vi "Example Write.vi"() -> ()   [LabVIEW 2010]
uses:
  C:/tf/play/labview/Tinkerforge.dll
  Tinkerforge.dll
panel:
  in  "stop":bool
  in  "uid":string="5556"
  in  "port":i32=4223
  in  "host":string="localhost"
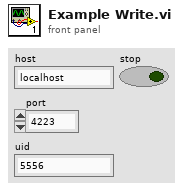
[diagram p1: front panel]
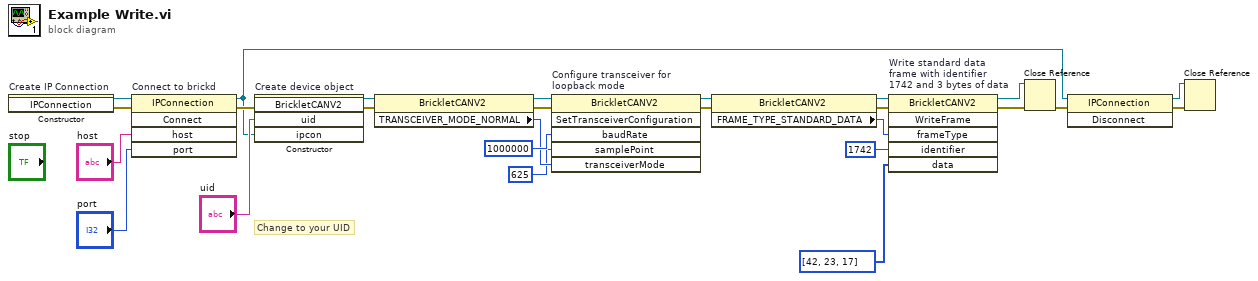
[diagram p0: block diagram]
diagram:
  # "Change to your UID"
  n1 = constructor on="Create IP Connection" class="IPConnection"() -> (reference out=w26:refnum<k24>, error out=w17:errorcluster)  [unwired: 3 in, 1 out]
  n2 = invoke on="Connect to brickd" class="IPConnection" method="Connect"(reference=w26, error in=w17, "host"="host", "port"="port") -> (reference out=w19:refnum<k24>, error out=w22:errorcluster)  [unwired: 1 in, 3 out]
  n3 = constructor on="Create device object" class="BrickletCANV2"(error in=w22, "uid"="uid", "ipcon"=w19) -> (reference out=w11:refnum<k24>, error out=w12:errorcluster)  [unwired: 2 in, 3 out]
  n4 = property class="BrickletCANV2"(reference=w11, error in=w12) -> (reference out=w9:refnum<k24>, error out=w10:errorcluster, "TRANSCEIVER_MODE_NORMAL"=w6:u8)
  n5 = invoke on="Configure transceiver for\nloopback mode" class="BrickletCANV2" method="SetTransceiverConfiguration"(reference=w9, error in=w10, "baudRate"=i64 1000000, "samplePoint"=625, "transceiverMode"=w6) -> (reference out=w2:refnum<k24>, error out=w1:errorcluster)  [unwired: 1 in, 4 out]
  n6 = property class="BrickletCANV2"(reference=w2, error in=w1) -> (reference out=w16:refnum<k24>, error out=w15:errorcluster, "FRAME_TYPE_STANDARD_DATA"=w14:u8)
  n7 = invoke on="Write standard data\nframe with identifier\n1742 and 3 bytes of data" class="BrickletCANV2" method="WriteFrame"(reference=w16, error in=w15, "frameType"=w14, "identifier"=i64 1742, "data"=u8[] [42, 23, 17]) -> (reference out=w3:refnum<k24>, error out=w4:errorcluster)  [unwired: 1 in, 4 out]
  n8 = Close Reference(reference=w3, error in (no error)=w4) -> (error out=w21:errorcluster)
  n9 = invoke class="IPConnection" method="Disconnect"(reference=w19, error in=w21) -> (reference out=w18:refnum<k24>, error out=w20:errorcluster)  [unwired: 1 in, 1 out]
  n10 = Close Reference(reference=w18, error in (no error)=w20) -> ()  [unwired: 1 out]
